vi "WhoAggregatesWhom.vi"(0 "reference":refnum<class "ClassRelationshipEdge.lvclass">, 5 "error in (no error)":errorcluster) -> (14 "reference out":refnum<class "ClassRelationshipEdge.lvclass">, 15 "AggregatesClass":refnum<class "AbstractNode.lvclass">, 16 "AggregatedClass":refnum<class "AbstractNode.lvclass">, 17 "CompositeAggregationUsed":bool, 19 "error out":errorcluster)   [LabVIEW 2012, in "ClassRelationshipEdge.lvclass"]
doc: "In which direction is the Triangle point, pointing."
uses:
  <resource>/Framework/Providers/Open_GDS/UML/ClassRelationshipEdge_class/ClassRelationshipEdge.lvclass
  <resource>/Framework/Providers/Open_GDS/UML/AbstractNode_class/AbstractNode.lvclass
  <resource>/Framework/Providers/Open_GDS/UML/ArrowHead_class/ArrowHead.lvclass
  <resource>/Framework/Providers/Open_GDS/UML/SegmentedLineEdge_class/SegmentedLineEdge.lvclass
  <resource>/Framework/Providers/Open_GDS/UML/AbstractEdge_class/AbstractEdge.lvclass
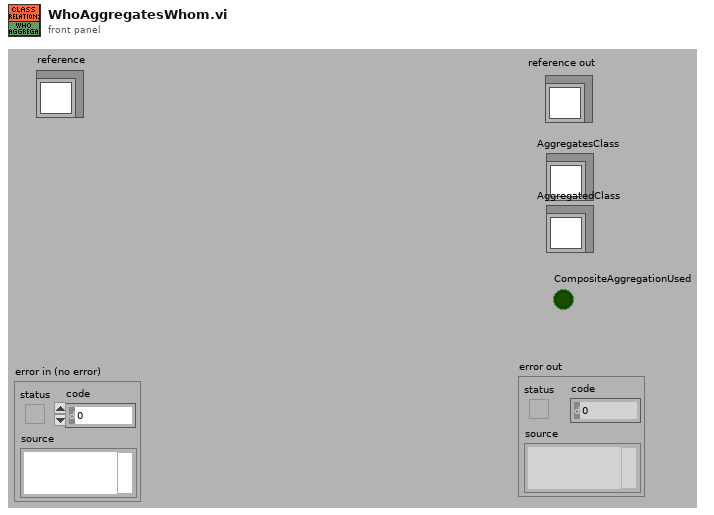
[diagram p1: front panel]
types:
  T1 = typedef "SegmentedLineEdge.lvclass/ObjectAttributes.ctl" = cluster{"lineStyle":refnum<class "LineStyle.lvclass">, "startArrowHead":refnum<class "ArrowHead.lvclass">, "endArrowHead":refnum<class "ArrowHead.lvclass">, "startLabel":string, "midLabel":string, "endLabel":string, "MidLabelOffset":T2, "SplitWire":bool}
  T2 = typedef "Point Point2D.ctl" = cluster{"x":dbl, "y":dbl}
  T3 = typedef "AbstractEdge.lvclass/ObjectAttributes.ctl" = cluster{"start":refnum<class "AbstractNode.lvclass">, "end":refnum<class "AbstractNode.lvclass">}
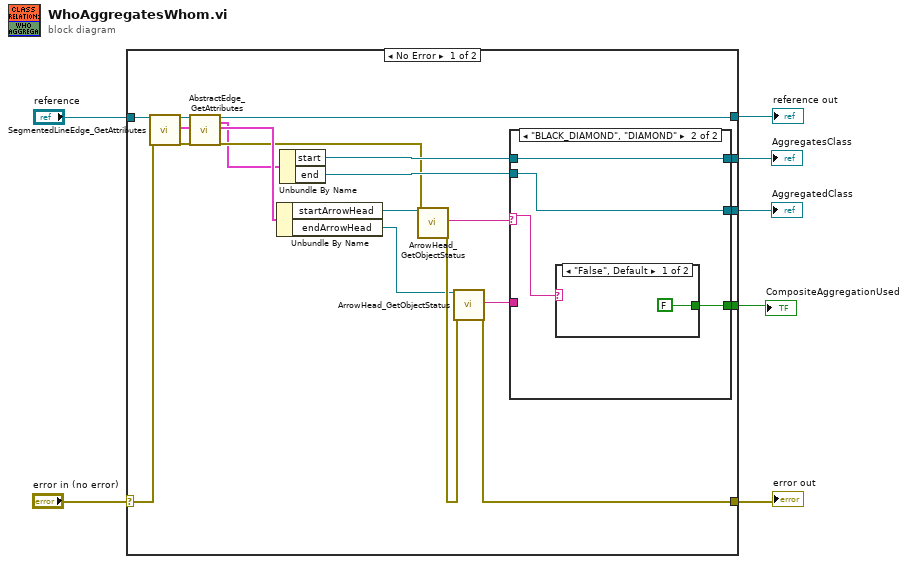
[diagram p0: block diagram]
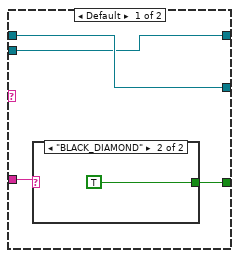
[diagram p2: hidden frame]
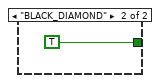
[diagram p4: hidden frame]
diagram:
  n1 = case shown="No Error" "error in (no error)" {
    selector: "error in (no error)" -> [w26 w38]
    tunnel: "reference" -> [w25 w39]
    tunnel: [w18 w38] -> w5
    tunnel: [w11 w39] -> w4
    tunnel: [w21 _] -> w3
    tunnel: [w20 _] -> w2
    tunnel: [w16 _] -> w1
    frame No Error {
      n2 = call <resource>:"SegmentedLineEdge_GetAttributes.vi"("reference in"=w25, "error in (no error)"=w26) -> ("reference out"=w14:refnum<class "ClassRelationshipEdge.lvclass">, "Data"=w15:T1, "error out"=w13:errorcluster)  [unwired: 14 in, 1 out]
      n3 = call <resource>:"AbstractEdge_GetAttributes.vi"("reference in"=w14, "error in (no error)"=w13) -> ("reference out"=w11:refnum<class "ClassRelationshipEdge.lvclass">, "Data"=w10:T3, "error out"=w12:errorcluster)  [unwired: 14 in, 1 out]
      n4 = Unbundle By Name(w15) -> ("startArrowHead"=w24:refnum<class "ArrowHead.lvclass">, "endArrowHead"=w17:refnum<class "ArrowHead.lvclass">)
      n5 = Unbundle By Name(w10) -> ("start"=w23:refnum<class "AbstractNode.lvclass">, "end"=w22:refnum<class "AbstractNode.lvclass">)
      n6 = call <resource>:"ArrowHead_GetObjectStatus.vi"("reference in"=w24, "error in (no error)"=w12) -> ("Object name"=w9:string, "error out"=w19:errorcluster)  [unwired: 1 in, 15 out]
      n7 = call <resource>:"ArrowHead_GetObjectStatus.vi"("reference in"=w17, "error in (no error)"=w19) -> ("Object name"=w8:string, "error out"=w18:errorcluster)  [unwired: 1 in, 15 out]
      n8 = case shown="\"BLACK_DIAMOND\", \"DIAMOND\"" w9 {
        selector: w9 -> [_ w34]
        tunnel: w23 -> [w28 w32]
        tunnel: w22 -> [w27 w33]
        tunnel: [w27 w32] -> w21
        tunnel: [w28 w33] -> w20
        tunnel: w8 -> [w30 _]
        tunnel: [w29 w35] -> w16
        frame Default {
          n9 = case shown="\"BLACK_DIAMOND\"" w30 {
            tunnel: [_ TRUE] -> w29
            frame Default {
            }
            frame "BLACK_DIAMOND" {
            }
          }
        }
        frame "BLACK_DIAMOND", "DIAMOND" {
          n10 = case shown="\"False\", Default" w34 {
            tunnel: [FALSE TRUE] -> w35
            frame "False", Default {
            }
            frame "BLACK_DIAMOND" {
            }
          }
        }
      }
    }
    frame Error {
    }
  }
  "reference out" <- w4
  "error out" <- w5
  "AggregatesClass" <- w3
  "AggregatedClass" <- w2
  "CompositeAggregationUsed" <- w1
